vi "File Path Globals.vi"() -> ()   [LabVIEW 2016]
panel:
  out "Filepath Array":string[](array[string])
  in  "FileName Array":string[](array[string])
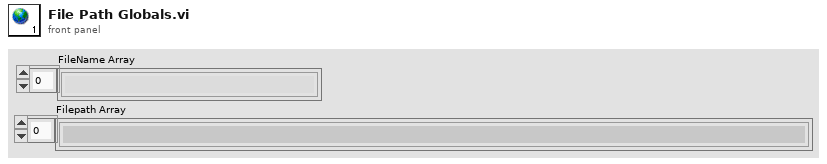
[diagram p1: front panel]
diagram:
